vi "N5765A_SetPSEnable.vi"(8 "error in (no error)":errorcluster, 9 "Enable Output (False)":bool, 11 "VISA resource name":refnum<visa-resource-name>="PowerSupply2") -> (0 "error out":errorcluster, 3 "VISA out":refnum<visa-resource-name>)   [LabVIEW 2015]
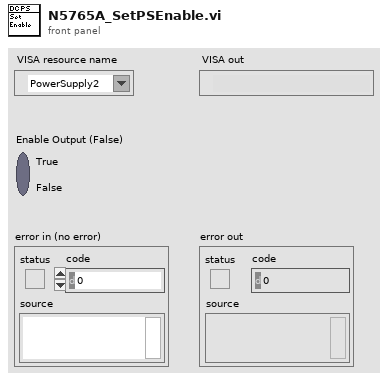
[diagram p1: front panel]
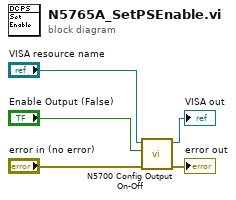
[diagram p0: block diagram]
diagram:
  n1 = call <instrlib>:"N5700 Config Output On-Off.vi"("error"="error in (no error)", "Output ON"="Enable Output (False)", "VISA"="VISA resource name") -> ("error out"=→"error out":errorcluster, "VISA out"=→"VISA out":refnum<visa-resource-name>)  [unwired: 4 in]
